vi "Show value.vi"(8 "error in (no error)":errorcluster caption="entrée d'erreur (pas d'erreur)", 11 "Maestro Control en entrée":refnum<class "Maestro Control.lvclass">) -> (0 "error out":errorcluster caption="sortie d'erreur", 3 "Maestro Control en sortie":refnum<class "Maestro Control.lvclass">)   [LabVIEW 2021, in "Maestro Control.lvclass"]
uses:
  Maestro Control.lvclass
  Maestro Control.lvclass/Maestro Control.ctl
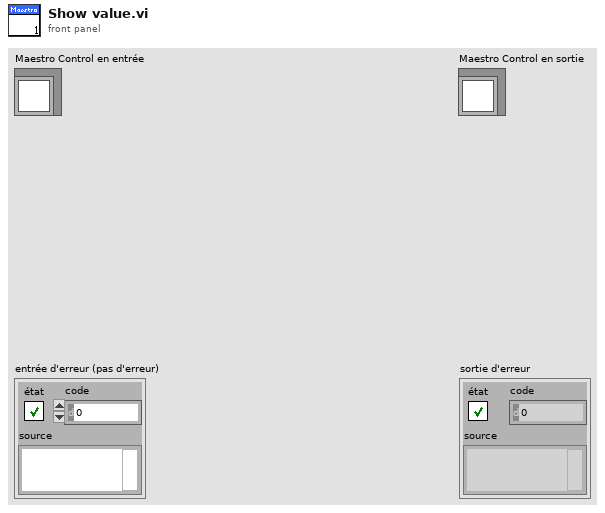
[diagram p1: front panel]
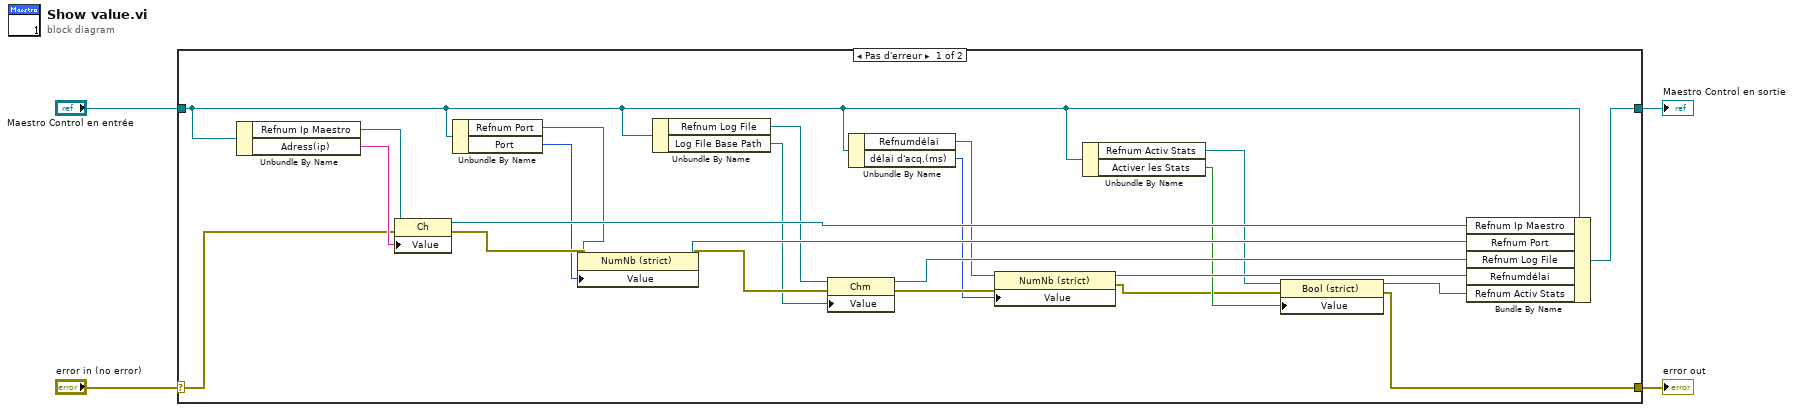
[diagram p0: block diagram]
diagram:
  n1 = case shown="Pas d'erreur" "error in (no error)" {
    selector: "error in (no error)" -> [w25 w29]
    tunnel: [w5 w29] -> w4
    tunnel: [w24 w28] -> w2
    tunnel: "Maestro Control en entrée" -> [w10 w28]
    frame No Error {
      n2 = Unbundle By Name(w10) -> ("Refnum Ip Maestro"=w23:refnum<vi>, "Adress(ip)"=w26:string)
      n3 = property class="Ch"(reference=w23, error in=w25, "Value"=w26) -> (reference out=w27:refnum<vi>, error out=w22:errorcluster)
      n4 = Unbundle By Name(w10) -> ("Refnum Port"=w21:refnum<vi>, "Port"=w20:i16)
      n5 = property class="NumNb (strict)"(reference=w21, error in=w22, "Value"=w20) -> (reference out=w19:refnum<vi>, error out=w18:errorcluster)
      n6 = Unbundle By Name(w10) -> ("Refnum Log File"=w16:refnum<vi>, "Log File Base Path"=w15:path)
      n7 = property class="Chm"(reference=w16, error in=w18, "Value"=w15) -> (reference out=w17:refnum<vi>, error out=w14:errorcluster)
      n8 = Unbundle By Name(w10) -> ("Refnumdélai"=w13:refnum<vi>, "délai d'acq.(ms)"=w12:i32)
      n9 = property class="NumNb (strict)"(reference=w13, error in=w14, "Value"=w12) -> (reference out=w11:refnum<vi>, error out=w6:errorcluster)
      n10 = Unbundle By Name(w10) -> ("Refnum Activ Stats"=w9:refnum<vi>, "Activer les Stats"=w8:bool)
      n11 = property class="Bool (strict)"(reference=w9, error in=w6, "Value"=w8) -> (reference out=w7:refnum<vi>, error out=w5:errorcluster)
      n12 = Bundle By Name(cluster=w10, "Refnum Ip Maestro"=w27, "Refnum Port"=w19, "Refnum Log File"=w17, "Refnumdélai"=w11, "Refnum Activ Stats"=w7) -> (w24:refnum<class "Maestro Control.lvclass">)
    }
    frame Error {
    }
  }
  "error out" <- w4
  "Maestro Control en sortie" <- w2
